vi "Set Name.vi"(8 "error in (no error)":errorcluster, 10 "Name":string, 11 "Node in":refnum<class "Node.lvclass">) -> (0 "error out":errorcluster, 3 "Node out":refnum<class "Node.lvclass">)   [LabVIEW 2020, in "PicoG-ParserLexer.lvlib" / "Node.lvclass"]
uses:
  Node.lvclass
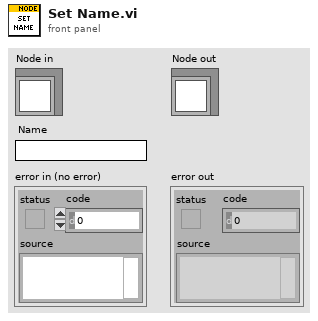
[diagram p1: front panel]
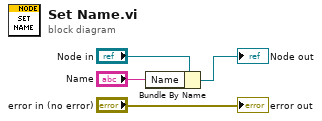
[diagram p0: block diagram]
diagram:
  n1 = Bundle By Name(cluster="Node in", "Name"="Name") -> (→"Node out":refnum<class "Node.lvclass">)
  "error out" <- "error in (no error)"
